vi "Create MetaData Element.vi"(6 "MetaData Parameters":T3, 7 "Channel Properties":T2, 8 "error in (no error)":errorcluster, 10 "Name":string, 11 "Refnum In":T1 format="%.0x") -> (0 "error out":errorcluster, 2 "Channel Refnum":T1 format="%.0x", 3 "Refnum Out":T1 format="%.0x")   [LabVIEW 2020, in "Instrument Addon Scripting API.lvlib"]
uses:
  Instrument Addon Scripting API.lvlib
  Shared Directory/MetaData Parameters.ctl
  Shared Directory/Protocol Data Type.ctl
  Shared Directory/Metadata Channel Type.ctl
  Shared Directory/Type Cast Type.ctl
  Shared Directory/Endian.ctl
  <vilib>/NI VeriStand/Custom Device API/Custom Device Item Ref.ctl
  TypeDefs/Channel Properties.ctl
  <vilib>/NI VeriStand/Custom Device API/Custom Device Channel.ctl
  <vilib>/NI VeriStand/Custom Device API/Custom Device Channel Type.ctl
  Shared Directory/FG Control.ctl
  Shared Directory/Constants.vi
  <vilib>/NI VeriStand/Custom Device API/NI VeriStand - Get Item Property.vi
  <vilib>/NI VeriStand/Custom Device API/Get Item Property (U32).vi
  <vilib>/NI VeriStand/Custom Device API/Get Item Property (String Array).vi
  <vilib>/NI VeriStand/Custom Device API/Get Item Property (String).vi
  <vilib>/NI VeriStand/Custom Device API/NI VeriStand - Set Item Property.vi
  <vilib>/NI VeriStand/Custom Device API/Set Item Property (U32).vi
  <vilib>/NI VeriStand/Custom Device API/Set Item Property (String Array).vi
  <vilib>/NI VeriStand/Custom Device API/NI VeriStand - Get Item Children.vi
  Shared Directory/Set Channel Value Table.vi
  <vilib>/NI VeriStand/Custom Device API/Set Item Property (String).vi
  Shared Directory/Instrument Addon Shared.lvlib
  <vilib>/NI VeriStand/Custom Device API/Custom Device API.lvlib
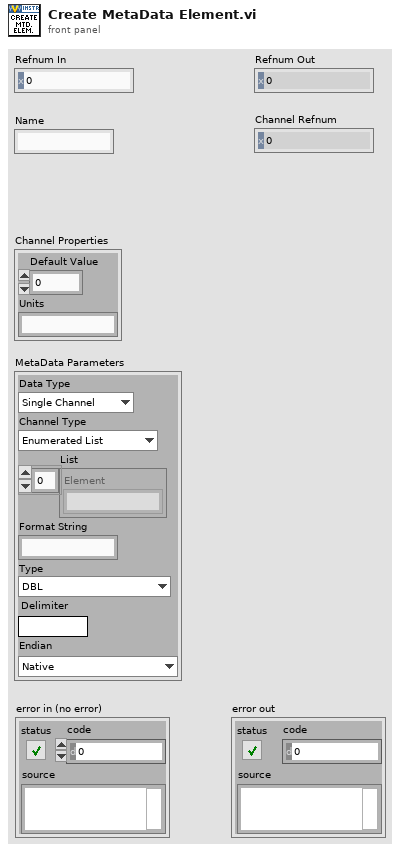
[diagram p1: front panel]
types:
  T1 = typedef "Custom Device API.lvlib/Custom Device Item Ref.ctl" = u64
  T2 = typedef "Instrument Addon Scripting API.lvlib/Channel Properties.ctl" = cluster{"Default Value":dbl, "Units":string}
  T3 = typedef "Instrument Addon Shared.lvlib/MetaData Parameters.ctl" = cluster{"Data Type":T4, "Channel Type":T5, "List":string[], "Format String":string, "Type":T6, "Delimiter":string, "Endian":T7}
  T4 = typedef "Instrument Addon Shared.lvlib/Protocol Data Type.ctl" = enum16{"Single Channel", "Array"}
  T5 = typedef "Instrument Addon Shared.lvlib/Metadata Channel Type.ctl" = enum16{"Enumerated List", "Format", "Type Cast"}
  T6 = typedef "Instrument Addon Shared.lvlib/Type Cast Type.ctl" = enum16{"DBL", "SGL", "U64", "U32", "U16", "U8", "I64", "I32", "I16", "I8"}
  T7 = typedef "Instrument Addon Shared.lvlib/Endian.ctl" = enum16{"Native", "Little", "Big"}
  T8 = typedef "Custom Device API.lvlib/Custom Device Channel Type.ctl" = enum16{"Input", "Output"}
  T9 = typedef "Instrument Addon Shared.lvlib/FG Control.ctl" = enum16{"Get", "Set"}
  T10 = typedef "Custom Device API.lvlib/Custom Device Channel.ctl" = cluster{"Type":T8, "Units":string, "Default Value":dbl, "Faultable":bool, "Scalable":bool}
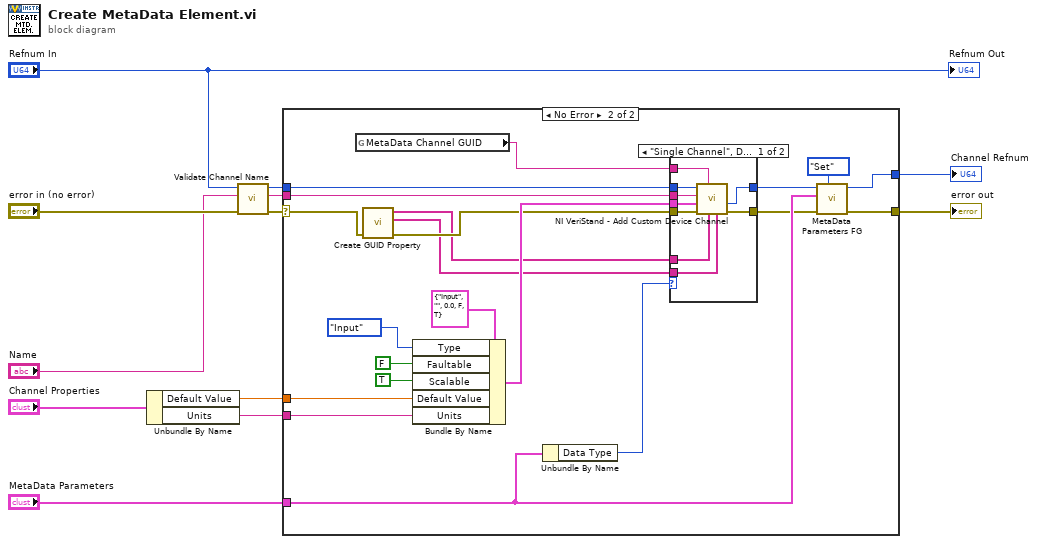
[diagram p0: block diagram]
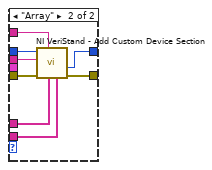
[diagram p3: hidden frame]
diagram:
  n1 = Unbundle By Name("Channel Properties") -> ("Default Value"=w9:dbl, "Units"=w8:string)
  n2 = call "Validate Channel Name.vi"("error in (no error)"="error in (no error)", "Name In"="Name", "Refnum In"="Refnum In") -> ("error out"=w5:errorcluster, "Name Out"=w4:string, "Refnum Out"=w3:T1)  [unwired: 6 in]
  n3 = case shown="No Error" w5 {
    selector: w5 -> [w13 w18]
    tunnel: w3 -> [w14 w35]
    tunnel: w4 -> [_ w34]
    tunnel: [w13 w21] -> w7
    tunnel: [w14 w22] -> w11
    tunnel: "MetaData Parameters" -> [_ w25]
    tunnel: w9 -> [_ w27]
    tunnel: w8 -> [_ w26]
    frame Error {
      # "Error case - Label is already in use"
    }
    frame No Error {
      n4 = global read "Constants.vi" "MetaData Channel GUID"() -> (w23:string)
      n5 = call "Create GUID Property.vi"("error in (no error)"=w18) -> ("error out"=w17:errorcluster, "property values"=w16:string[], "property names"=w15:string[])  [unwired: 8 in]
      n6 = Bundle By Name(cluster=T10 {"Type"=enum."Input", "Units"="", "Default Value"=0.0, "Faultable"=FALSE, "Scalable"=TRUE} ("Channel"), "Type"=Custom_Device_Channel_Type."Input", "Faultable"=FALSE, "Scalable"=TRUE, "Default Value"=w27, "Units"=w26) -> (w28:T10)
      n7 = Unbundle By Name(w25) -> ("Data Type"=w24:T4)
      n8 = case shown="\"Single Channel\", Default" w24 {
        tunnel: w23 -> [w39 w48]
        tunnel: w35 -> [w44 w49]
        tunnel: w34 -> [w43 w47]
        tunnel: w17 -> [w42 w52]
        tunnel: [w41 w51] -> w20
        tunnel: [w38 w50] -> w19
        tunnel: w28 -> [w40 _]
        tunnel: w16 -> [w36 w46]
        tunnel: w15 -> [w37 w45]
        frame "Single Channel", Default {
          n9 = call <vilib>:"NI VeriStand - Add Custom Device Channel.vi"("Property Values"=w36, "Property names"=w37, "GUID (Default Channel)"=w39, "error in (no error)"=w42, "Channel"=w40, "Channel Name"=w43, "Parent Ref in"=w44) -> ("error out"=w41:errorcluster, "Channel Ref"=w38:T1)  [unwired: 1 in, 2 out]
        }
        frame "Array" {
          n10 = call <vilib>:"NI VeriStand - Add Custom Device Section.vi"("Property Values"=w46, "Property names"=w45, "GUID (Default Section)"=w48, "error in (no error)"=w52, "Section Name"=w47, "Parent Ref in"=w49) -> ("error out"=w51:errorcluster, "Section Ptr"=w50:T1)  [unwired: 2 in, 2 out]
        }
      }
      n11 = call "MetaData Parameters FG.vi"("Action"=FG_Control."Set", "error in (no error)"=w20, "MetaData Parameters"=w25, "Item Ref in"=w19) -> ("error out"=w21:errorcluster, "Item Ref out"=w22:T1)  [unwired: 5 in, 1 out]
    }
  }
  "Channel Refnum" <- w11
  "error out" <- w7
  "Refnum Out" <- "Refnum In"
